vi "Pack to Any.vi"(8 "error in":errorcluster, 9 "Data To Pack":T3={"Frequency"=0.0, "Amplitude"=1.0}, 10 "Message Type":string, 11 "gRPCid in":T2) -> (0 "error out":errorcluster, 2 "Any":T1, 3 "gRPCid out":u64)   [LabVIEW 2020]
uses:
  Measurement Configuration.ctl
  <vilib>/gRPC/LabVIEW gRPC Library/Shared/grpcId.ctl
  <vilib>/gRPC/LabVIEW gRPC Library/Shared/Any.ctl
  <vilib>/AdvancedString/1D String Array to Delimited String.vi
  <vilib>/gRPC/LabVIEW gRPC Library/grpc-lvsupport-release.lvlib
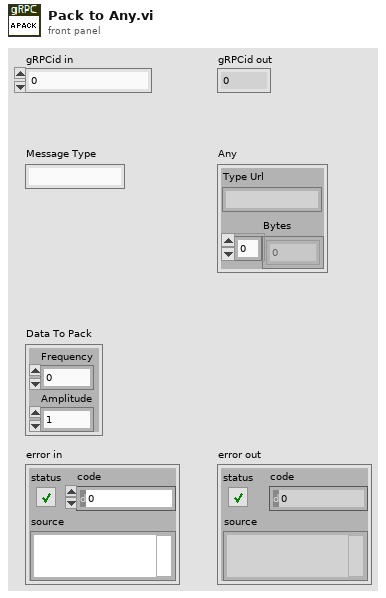
[diagram p1: front panel]
types:
  T1 = typedef "grpc-lvsupport-release.lvlib/Any.ctl" = cluster{"Type Url":string, "Bytes":u8[]}
  T2 = typedef "grpc-lvsupport-release.lvlib/grpcId.ctl" = u64
  T3 = typedef "Measurement Configuration.ctl" = cluster{"Frequency":dbl, "Amplitude":dbl}
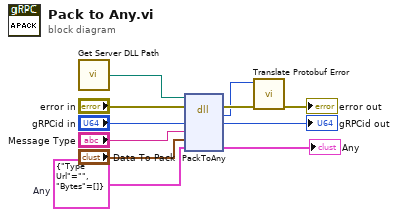
[diagram p0: block diagram]
diagram:
  w4 = T1 {"Type Url"="", "Bytes"=[]}  # Any
  n1 = call <vilib>:"Get Server DLL Path.vi"() -> ("Server dll path"=w9:path)
  n2 = dll-call lib="?" fn="PackToAny"(path in=w9, error in="error in", "gRPCId"="gRPCid in", "messageType"="Message Type", "value"="Data To Pack", "any"=w4) -> (error out=w10:errorcluster, "return type"=w1:i32, "gRPCId"=→"gRPCid out":u64, "any"=→"Any":T1)  [unwired: 3 in, 1 out]
  n3 = call <vilib>:"Translate Protobuf Error.vi"("error in"=w10, "Error Code"=w1) -> ("error out"=→"error out":errorcluster)  [unwired: 9 in]
